vi "Get Comms Loop Next State.vi"(8 "error in (no error)":errorcluster) -> (0 "error out":errorcluster, 3 "Data":variant, 5 "Command":T1)   [LabVIEW 2019]
uses:
  Controls/Comms Loop States.ctl
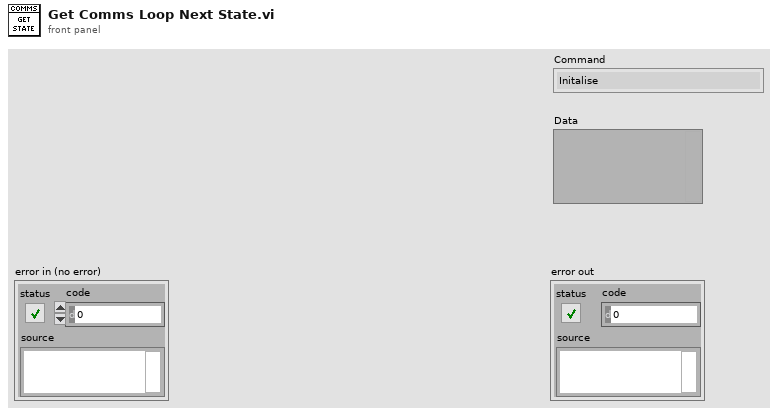
[diagram p1: front panel]
types:
  T1 = typedef "Comms Loop States.ctl" = enum16{"Initalise", "User Event", "HEART_BEAT", "SEND_LOG_FILE_NAME", "Clear Log File Names", "SEND_LOG_FILE_CHUNK", "SEND_LOG_FILE_SIZE", "SEND_SD_CARD_INFO", "SEND_BATTERY_INFO", "SEND_LOGGING_PERIOD", "SEND_RTC_TIME", "SEND_CURRENT_MEASUREMENTS", "ERROR_MSG", "Clear Error Messages", "Send Message", "Idle", "Sensor Connected", "Sensor Disconnected", "Set Page Displayed", "Set Connected Sensor Type", "UI: Update Sensor Type", "UI: Update Log List", "Reset Log File Transfer", "SEND_WIFI_DETAILS", "Complete Transfer"}
  T2 = typedef "Comms Loop State Controller Message.ctl" = cluster{"Command":T1, "Data":variant}
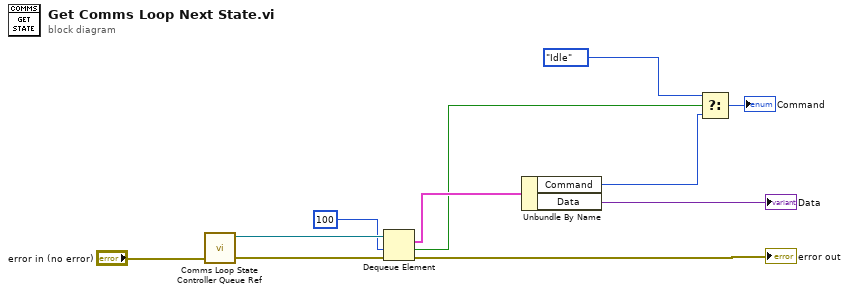
[diagram p0: block diagram]
diagram:
  n1 = call "Comms Loop State Controller Queue Ref.vi"("error in (no error)"="error in (no error)") -> ("error out"=w7:errorcluster, "queue out"=w6:refnum<queue>)  [unwired: 9 in]
  n2 = Dequeue Element(queue=w6, timeout in ms (-1)=100, error in (no error)=w7) -> (element=w10:T2, timed out?=w5:bool, error out=→"error out":errorcluster)  [unwired: 1 out]
  n3 = Unbundle By Name(w10) -> ("Command"=w4:T1, "Data"=→"Data":variant)
  n4 = Select(t=Comms_Loop_States."Idle", s=w5, f=w4) -> (s? t:f=→"Command":T1)
